vi "Compute Distance Glenn.vi"(8 "Y Image Resolution":i32, 9 "X Image Resolution":i32, 10 "Target Corners":T1, 11 "Camera Type":enum16{"206", "1011"}(ring)) -> (2 "Target Center (-1 to 1)":cluster{"X":dbl, "Y":dbl}, 3 "Distance (ft)":dbl)   [LabVIEW 2011]
doc: "Using the camera lens information and the real world width of the target, determine the distance to the target."
panel:
  in  "Camera view angle":dbl[](array[numeric])=[48.0, 43.5]
  # "Axis 206\nAxis M1011"
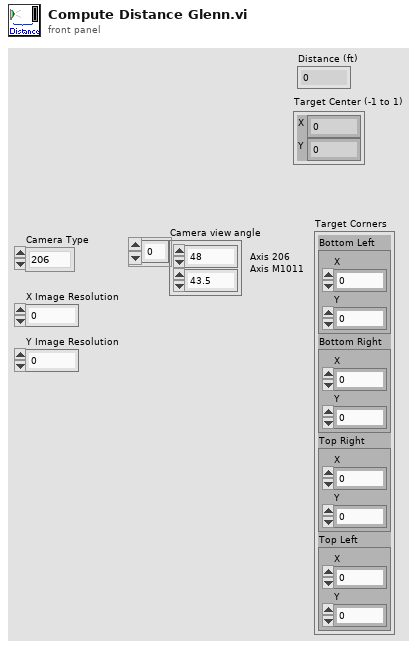
[diagram p1: front panel]
types:
  T1 = cluster{"Bottom Left":cluster{"X":dbl, "Y":dbl}, "Bottom Right":cluster{"X":dbl, "Y":dbl}, "Top Right":cluster{"X":dbl, "Y":dbl}, "Top Left":cluster{"X":dbl, "Y":dbl}}
  T2 = cluster{"X Image Resolution":i32, "Y Image Resolution":i32}
  T3 = cluster{"X Image Resolution":dbl, "Y Image Resolution":dbl}
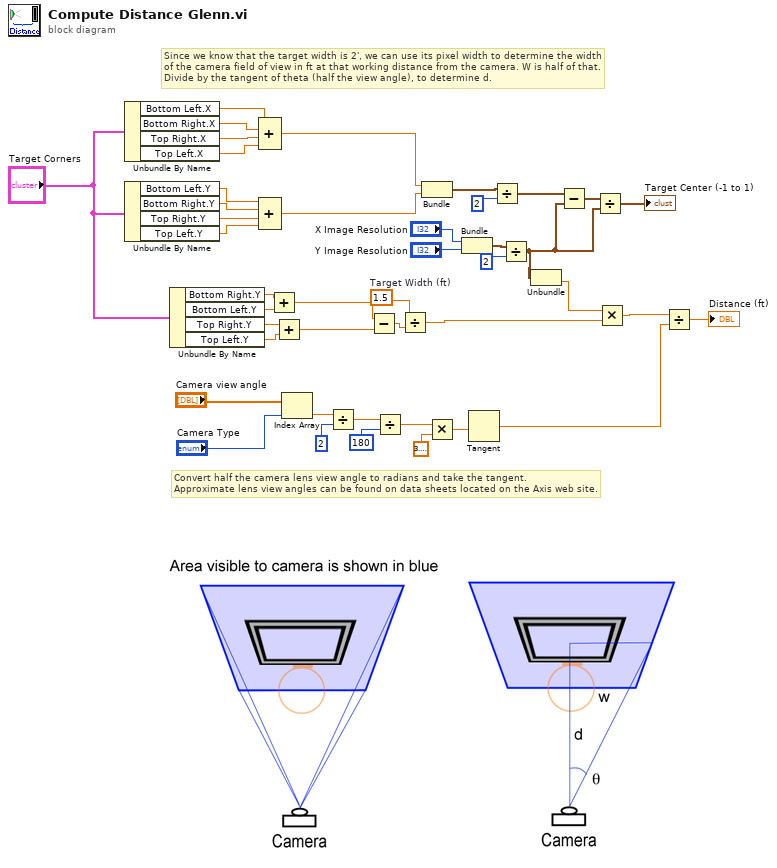
[diagram p0: block diagram]
diagram:
  w31 = 1.5  # Target Width (ft)
  # "Convert half the camera lens view angle to radians and take the tangent.\nApproximate lens view angles can be found on data sheets located on the Axis web site."
  # "Since we know that the target width is 2', we can use its pixel width to determine the width\nof the camera field of view in ft at that working distance from the camera. W is half of that.\nDivide by the tangent of theta (half the view angle), to determine d."
  n1 = Unbundle By Name("Target Corners") -> ("Bottom Left.X"=w19:dbl, "Bottom Right.X"=w18:dbl, "Top Right.X"=w17:dbl, "Top Left.X"=w16:dbl)
  n2 = Unbundle By Name("Target Corners") -> ("Bottom Left.Y"=w14:dbl, "Bottom Right.Y"=w13:dbl, "Top Right.Y"=w12:dbl, "Top Left.Y"=w11:dbl)
  n3 = Unbundle By Name("Target Corners") -> ("Bottom Right.Y"=w7:dbl, "Bottom Left.Y"=w8:dbl, "Top Right.Y"=w5:dbl, "Top Left.Y"=w4:dbl)
  n4 = Compound Arithmetic op=ADD(w19, w18, w17, w16) -> (w9:dbl)
  n5 = Compound Arithmetic op=ADD(w14, w13, w12, w11) -> (w10:dbl)
  n6 = Add(x=w7, y=w8) -> (x+y=w6:dbl)
  n7 = Add(x=w5, y=w4) -> (x+y=w3:dbl)
  n8 = Index Array(array="Camera view angle", index="Camera Type") -> (element=w39:dbl)
  n9 = Divide(x=w39, y=2) -> (x/y=w36:dbl)
  n10 = Subtract(x=w6, y=w3) -> (x-y=w33:dbl)
  n11 = Divide(x=w36, y=180) -> (x/y=w35:dbl)
  n12 = Divide(x=w31, y=w33) -> (x/y=w32:dbl)
  n13 = Bundle(w9, w10) -> (w2:cluster{dbl, dbl})  [unwired: 1 in]
  n14 = Multiply(x=w35, y=3.141592653589793) -> (x*y=w37:dbl)
  n15 = Bundle("X Image Resolution"="X Image Resolution", "Y Image Resolution"="Y Image Resolution") -> (w27:T2)  [unwired: 1 in]
  n16 = Tangent(1:w37) -> (0:w43:dbl)
  n17 = Divide(x=w2, y=2) -> (x/y=w25:cluster{dbl, dbl})
  n18 = Divide(x=w27, y=2) -> (x/y=w21:T3)
  n19 = Unbundle(w21) -> ("Y Image Resolution"=w20:dbl)  [unwired: 1 out]
  n20 = Subtract(x=w25, y=w21) -> (x-y=w24:cluster{dbl, dbl})
  n21 = Divide(x=w24, y=w21) -> (x/y=→"Target Center (-1 to 1)":cluster{dbl, dbl})
  n22 = Multiply(x=w20, y=w32) -> (x*y=w22:dbl)
  n23 = Divide(x=w22, y=w43) -> (x/y=→"Distance (ft)":dbl)
